vi "Add Error Channel Manager.vi"(8 "error in (no error)":errorcluster, 9 "String to Append":string, 10 "Error":T1, 11 "Insert Error":bool=TRUE) -> (0 "error out":errorcluster)   [LabVIEW 2021, in "CIFChannelMng.lvclass"]
uses:
  CIFChannelMng.lvclass
  typedef/Errors Channel Manager.ctl
  <vilib>/CIF Foundation/CIF Utilities/Errors/Errors_CIF_U.lvlib
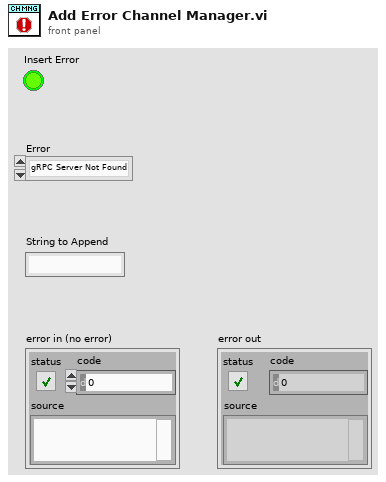
[diagram p1: front panel]
types:
  T1 = typedef "CIFChannelMng.lvclass/Errors Channel Manager.ctl" = enum16{"gRPC Server Not Found", "Duplicate Channel", "Missing Channel", "Incorrect Type", "Flatten Error", "Unflatten Data", "Channel Length", "Plugin Connection", "gRPC Server Connection", "FIFO Unflatten", "Required Override", "Remove Not Found"}
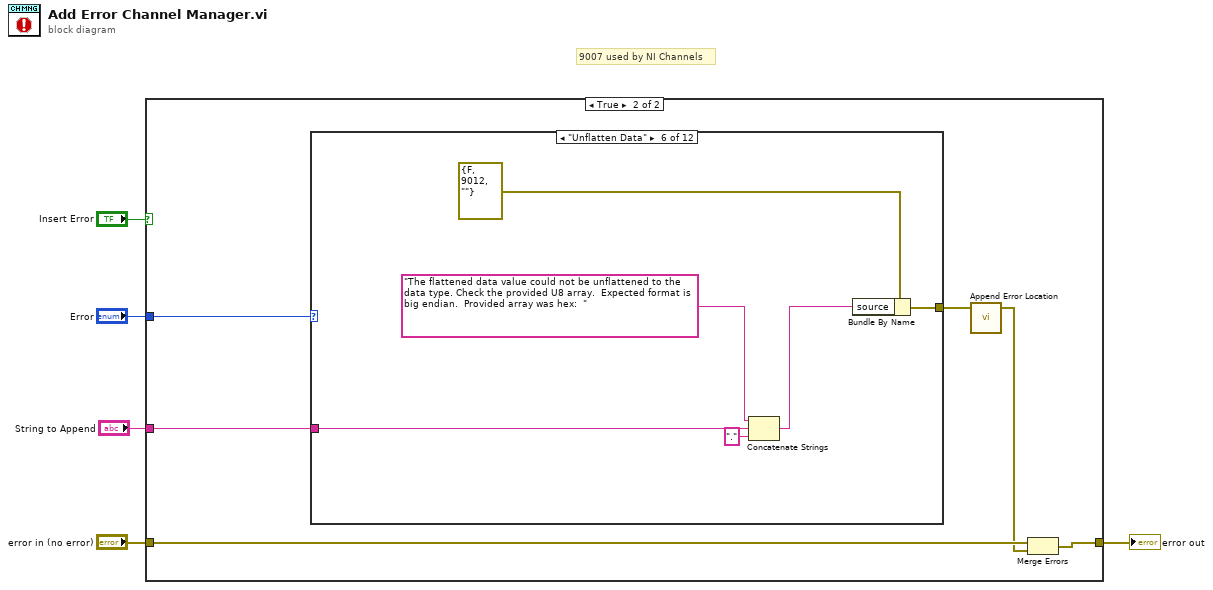
[diagram p0: block diagram]
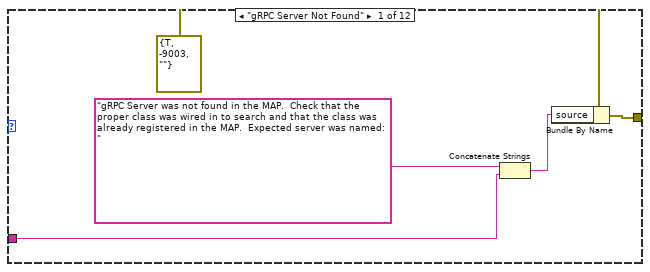
[diagram p3: hidden frame]
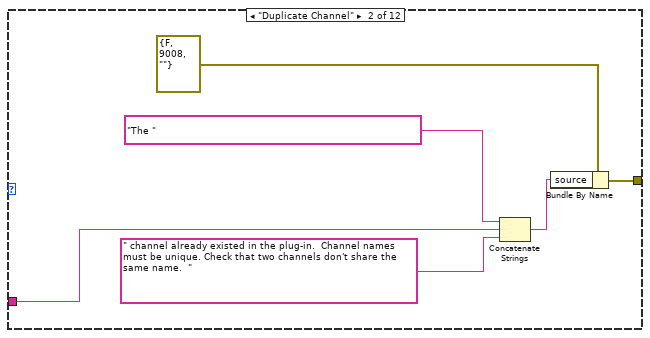
[diagram p4: hidden frame]
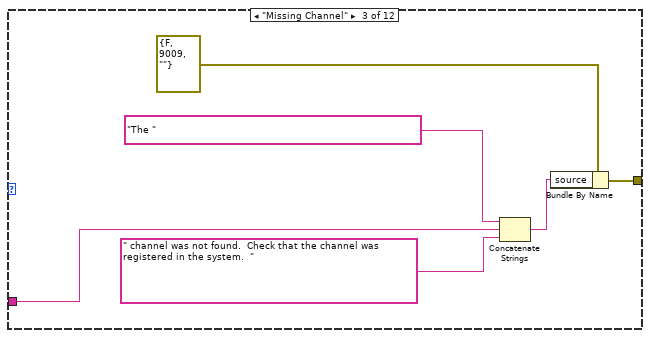
[diagram p5: hidden frame]
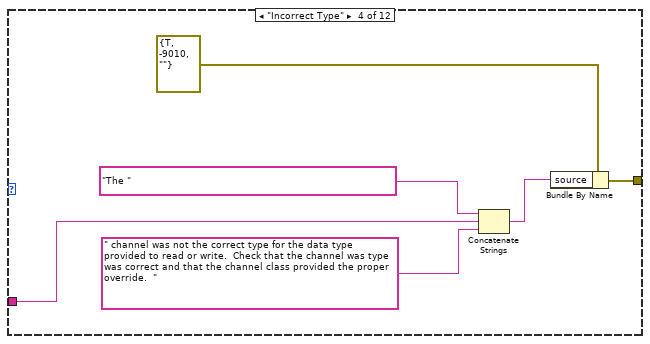
[diagram p6: hidden frame]
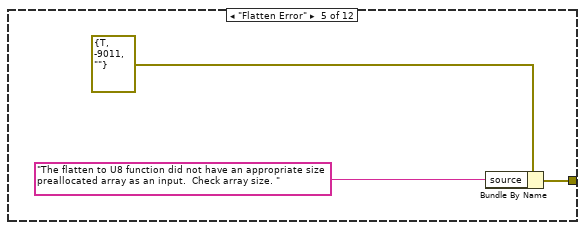
[diagram p7: hidden frame]
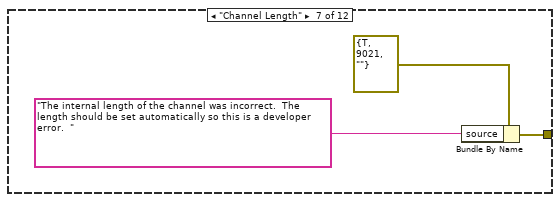
[diagram p8: hidden frame]
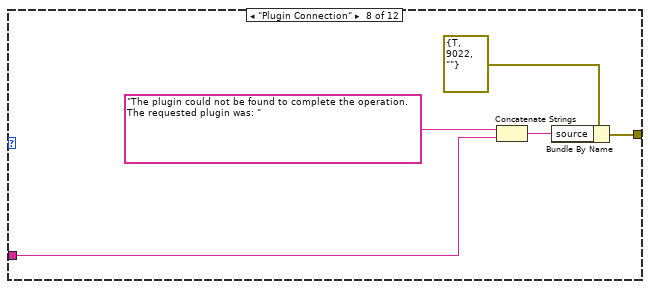
[diagram p9: hidden frame]
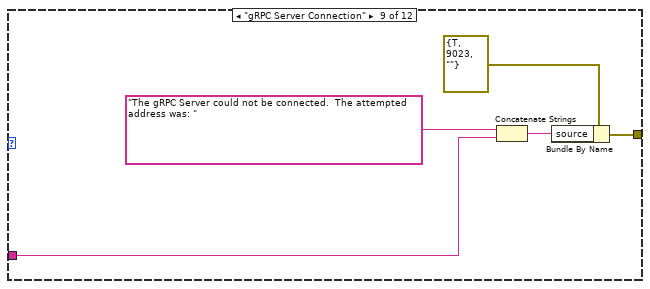
[diagram p10: hidden frame]
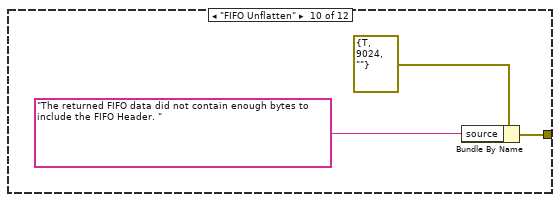
[diagram p11: hidden frame]
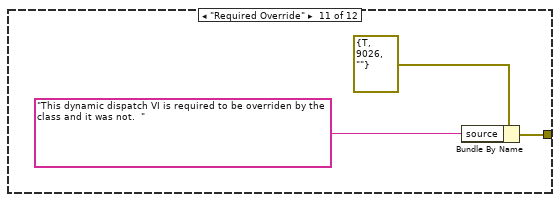
[diagram p12: hidden frame]
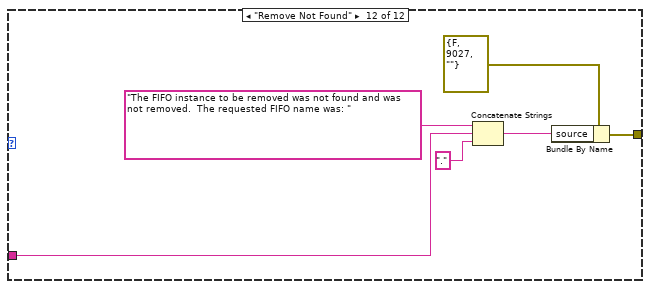
[diagram p13: hidden frame]
diagram:
  # "9007 used by NI Channels"
  n1 = case shown="True" "Insert Error" {
    tunnel: [w6 w9] -> w4
    tunnel: "error in (no error)" -> [w6 w10]
    tunnel: "Error" -> [_ w12]
    tunnel: "String to Append" -> [_ w11]
    frame False {
    }
    frame True {
      n2 = case shown="\"Unflatten Data\"" w12 {
        tunnel: w11 -> [w14 w20 w24 w30 _ w41 _ w48 w53 _ _ w66]
        tunnel: [w16 w22 w28 w34 w37 w43 w46 w51 w56 w59 w62 w68] -> w8
        frame "gRPC Server Not Found" {
          n3 = Concatenate Strings("gRPC Server was not found in the MAP.  Check that the proper class was wired in to search and that the class was already registered in the MAP.  Expected server was named:  " ("source"), w14) -> (w15:string)
          n4 = Bundle By Name(cluster=errorcluster {"status"=TRUE, "code"=-9003, "source"=""} ("Invalid ID"), "source"=w15) -> (w16:errorcluster)
        }
        frame "Duplicate Channel" {
          n5 = Concatenate Strings("The " ("source"), w20, " channel already existed in the plug-in.  Channel names must be unique. Check that two channels don't share the same name.  " ("source")) -> (w21:string)
          n6 = Bundle By Name(cluster=errorcluster {"status"=FALSE, "code"=9008, "source"=""} ("Invalid ID"), "source"=w21) -> (w22:errorcluster)
        }
        frame "Missing Channel" {
          n7 = Concatenate Strings("The " ("source"), w24, " channel was not found.  Check that the channel was registered in the system.  " ("source")) -> (w27:string)
          n8 = Bundle By Name(cluster=errorcluster {"status"=FALSE, "code"=9009, "source"=""} ("Invalid ID"), "source"=w27) -> (w28:errorcluster)
        }
        frame "Incorrect Type" {
          n9 = Concatenate Strings("The " ("source"), w30, " channel was not the correct type for the data type provided to read or write.  Check that the channel was type was correct and that the channel class provided the proper override.  " ("source")) -> (w31:string)
          n10 = Bundle By Name(cluster=errorcluster {"status"=TRUE, "code"=-9010, "source"=""} ("Invalid ID"), "source"=w31) -> (w34:errorcluster)
        }
        frame "Flatten Error" {
          n11 = Bundle By Name(cluster=errorcluster {"status"=TRUE, "code"=-9011, "source"=""} ("Invalid ID"), "source"="The flatten to U8 function did not have an appropriate size preallocated array as an input.  Check array size. ") -> (w37:errorcluster)
        }
        frame "Unflatten Data" {
          n12 = Concatenate Strings("The flattened data value could not be unflattened to the data type. Check the provided U8 array.  Expected format is big endian.  Provided array was hex:  " ("source"), w41, "." ("string")) -> (w39:string)
          n13 = Bundle By Name(cluster=errorcluster {"status"=FALSE, "code"=9012, "source"=""} ("Invalid ID"), "source"=w39) -> (w43:errorcluster)
        }
        frame "Channel Length" {
          n14 = Bundle By Name(cluster=errorcluster {"status"=TRUE, "code"=9021, "source"=""} ("Invalid ID"), "source"="The internal length of the channel was incorrect.  The length should be set automatically so this is a developer error.  ") -> (w46:errorcluster)
        }
        frame "Plugin Connection" {
          n15 = Concatenate Strings("The plugin could not be found to complete the operation.  The requested plugin was: " ("source"), w48) -> (w49:string)
          n16 = Bundle By Name(cluster=errorcluster {"status"=TRUE, "code"=9022, "source"=""} ("Invalid ID"), "source"=w49) -> (w51:errorcluster)
        }
        frame "gRPC Server Connection" {
          n17 = Concatenate Strings("The gRPC Server could not be connected.  The attempted address was: " ("source"), w53) -> (w54:string)
          n18 = Bundle By Name(cluster=errorcluster {"status"=TRUE, "code"=9023, "source"=""} ("Invalid ID"), "source"=w54) -> (w56:errorcluster)
        }
        frame "FIFO Unflatten" {
          n19 = Bundle By Name(cluster=errorcluster {"status"=TRUE, "code"=9024, "source"=""} ("Invalid ID"), "source"="The returned FIFO data did not contain enough bytes to include the FIFO Header. ") -> (w59:errorcluster)
        }
        frame "Required Override" {
          n20 = Bundle By Name(cluster=errorcluster {"status"=TRUE, "code"=9026, "source"=""} ("Invalid ID"), "source"="This dynamic dispatch VI is required to be overriden by the class and it was not.  ") -> (w62:errorcluster)
        }
        frame "Remove Not Found" {
          n21 = Concatenate Strings("The FIFO instance to be removed was not found and was not removed.  The requested FIFO name was: " ("source"), w66, "." ("string")) -> (w64:string)
          n22 = Bundle By Name(cluster=errorcluster {"status"=FALSE, "code"=9027, "source"=""} ("Invalid ID"), "source"=w64) -> (w68:errorcluster)
        }
      }
      n23 = call <vilib>:"Append Error Location.vi"("error in (no error)"=w8) -> ("error out"=w7:errorcluster)  [unwired: 4 in]
      n24 = Merge Errors(w10, w7) -> (w9:errorcluster)
    }
  }
  "error out" <- w4
